vi "Convert PNG to VIs.vi"(8 "error in (no error)":errorcluster) -> (0 "error out":errorcluster, 3 "directory copy":path)   [LabVIEW 2015]
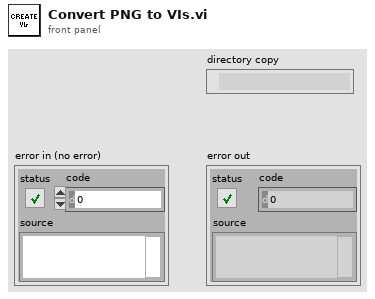
[diagram p1: front panel]
types:
  T1 = cluster{"left":i16, "top":i16, "right":i16, "bottom":i16}
  T2 = typedef "imagedata.ctl" = cluster{"image type":i32, "image depth":i32, "image":u8[], "mask":u8[], "colors":u32[], "Rectangle":cluster{"left":i16, "top":i16, "right":i16, "bottom":i16}}
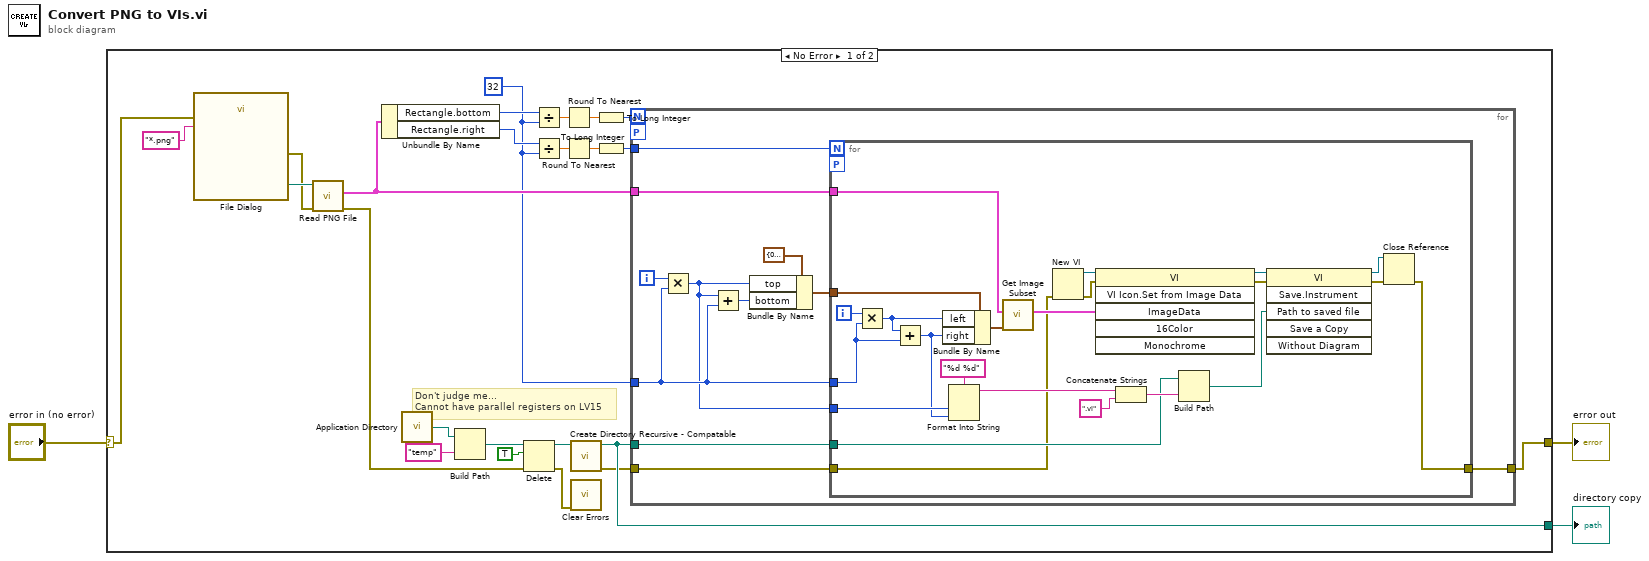
[diagram p0: block diagram]
diagram:
  n1 = case shown="No Error" "error in (no error)" {
    selector: "error in (no error)" -> [w9 w62]
    tunnel: [w6 _] -> w3
    tunnel: [w8 w62] -> w1
    frame No Error {
      w15 = i16 32 ("y")
      # "Don't judge me...\nCannot have parallel registers on LV15"
      n2 = call "File Dialog"("error in"=w9, "pattern (all files)"="*.png") -> ("selected path"=w22:path, "error out"=w11:errorcluster)  [unwired: 10 in, 2 out]
      n3 = call <vilib>:"Read PNG File.vi"("error in (no error)"=w11, "path to PNG file"=w22) -> ("error out"=w10:errorcluster, "image data"=w27:T2)  [unwired: 7 in, 1 out]
      n4 = Unbundle By Name(w27) -> ("Rectangle.bottom"=w26:i16, "Rectangle.right"=w16:i16)
      n5 = call <vilib>:"Application Directory.vi"() -> ("Application Directory"=w19:path)
      n6 = Build Path(base path=w19, name or relative path="temp") -> (appended path=w20:path)
      n7 = Delete(path (use dialog)=w20, entire hierarchy (F)=TRUE, error in=w10) -> (deleted path=w7:path, error out=w4:errorcluster)  [unwired: 2 in, 1 out]
      n8 = Divide(x=w26, y=w15) -> (x/y=w24:dbl)
      n9 = Divide(x=w16, y=w15) -> (x/y=w25:dbl)
      n10 = Round To Nearest(number=w24) -> (nearest integer value=w14:dbl)
      n11 = Round To Nearest(number=w25) -> (nearest integer value=w23:dbl)
      n12 = call "Create Directory Recursive - Compatable.vi"("directory"=w7) -> ("error out"=w5:errorcluster, "directory copy"=w6:path)  [unwired: 8 in, 1 out]
      n13 = call <vilib>:"Clear Errors.vi"("error in (no error)"=w4) -> ()  [unwired: 5 in, 2 out]
      n14 = To Long Integer(number=w14) -> (32bit integer=w13:i32)
      n15 = To Long Integer(number=w23) -> (32bit integer=w12:i32)
      n16 = for {
        N: w13 -> [_]
        tunnel: w27 -> [w38]
        tunnel: w12 -> [w37]
        tunnel: w15 -> [w34]
        tunnel: w6 -> [w31]
        workers-P: _ -> [_]
        tunnel: w5 -> [w29]
        tunnel: [w28] -> w8
        i -> [w35]
        n17 = Multiply(x=w35, y=w34) -> (x*y=w32:i32)
        n18 = Add(x=w32, y=w34) -> (x+y=w33:i32)
        n19 = Bundle By Name(cluster=T1 {"left"=0, "top"=0, "right"=0, "bottom"=0} ("subset rect"), "top"=w32, "bottom"=w33) -> (w36:T1)
        n20 = for {
          N: w37 -> [_]
          tunnel: w36 -> [w61]
          tunnel: w38 -> [w60]
          tunnel: w34 -> [w58]
          tunnel: w32 -> [w45]
          tunnel: w31 -> [w42]
          workers-P: _ -> [_]
          tunnel: w29 -> [w41]
          tunnel: [w39] -> w28
          i -> [w59]
          n21 = Multiply(x=w59, y=w58) -> (x*y=w44:i32)
          n22 = Add(x=w44, y=w58) -> (x+y=w43:i32)
          n23 = Bundle By Name(cluster=w61, "left"=w44, "right"=w43) -> (w48:T1)
          n24 = Format Into String(format string="%d %d", w45, w43) -> (resulting string=w46:string)  [unwired: 2 in, 1 out]
          n25 = call <vilib>:"Get Image Subset.vi"("subset rect"=w48, "image data"=w60) -> ("image subset"=w56:T2)  [unwired: 4 in, 1 out]
          n26 = New VI(8:w41) -> (0:w40:errorcluster, 3:w57:refnum<vi>)  [unwired: 6 in]
          n27 = invoke class="VI" method="VI Icon.Set from Image Data"(reference=w57, error in=w40, "ImageData"=w56) -> (reference out=w55:refnum<vi>, error out=w51:errorcluster)  [unwired: 3 in, 4 out]
          n28 = Concatenate Strings(w46, ".vi" ("string")) -> (w54:string)
          n29 = Build Path(base path=w42, name or relative path=w54) -> (appended path=w52:path)
          n30 = invoke class="VI" method="Save.Instrument"(reference=w55, error in=w51, "Path to saved file"=w52) -> (reference out=w50:refnum<vi>, error out=w49:errorcluster)  [unwired: 3 in, 4 out]
          n31 = Close Reference(reference=w50, error in (no error)=w49) -> (error out=w39:errorcluster)
        }
      }
    }
    frame Error {
    }
  }
  "error out" <- w1
  "directory copy" <- w3
